vi "Read Data.vi"(0 "comm interface in":refnum<class "Pixy Com.lvclass">, 5 "bytes to read":i32, 11 "error in":errorcluster) -> (4 "comm interface out":refnum<class "Pixy Com.lvclass">, 6 "data":u8[](array[numeric]), 15 "error out":errorcluster)   [LabVIEW 2018, in "Pixy2.lvlib" / "Pixy Com.lvclass"]
uses:
  Pixy Com.lvclass
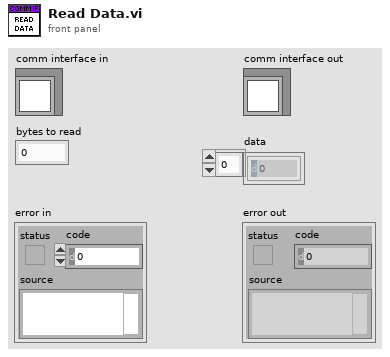
[diagram p1: front panel]
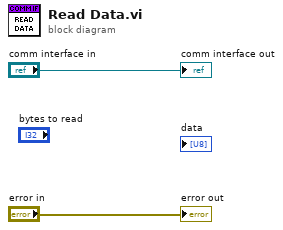
[diagram p0: block diagram]
diagram:
  "error out" <- "error in"
  "comm interface out" <- "comm interface in"
